vi "SeCrTs-DI Indexing.vi"(9 "data":T1={"AO config"=[], "AI config"=[], "DI config"=[], "DO config"=[], "TC config"=[], "ACC config"=[], "SG config"=[], "Strain Gauge Settings"={"poisson ratio"=0.3, "nominal gage resistance"=120.0, "gage factor"=2.08}, "Bridge Settings"={"voltage excitation value"=3.3, "voltage excitation source"=10200, "initial bridge voltage"=0.0, "lead wire resistance"=1.7, "strain configuration"=10271}, "Sample Rate"={"AI Sample Rate"=[], "AO Sample Rate"=[], "DI Sample Rate"=[], "TC Sample Rate"=[], "DO Sample Rate"=[], "SG Sample Rate"=[], "ACC Sample Rate"=[]}} {"Bridge Settings"."strain configuration" items=["Full Bridge I"=10183, "Full Bridge II"=10184, "Full Bridge III"=10185, "Half Bridge I"=10188, "Half Bridge II"=10189, "Quarter Bridge I"=10271, "Quarter Bridge II"=10272]; "Bridge Settings"."voltage excitation source" items=["Internal"=10200, "External"=10167, "None"=10230]; "ACC config"."Terminal configuration" items=["default"=-1, "RSE"=10083, "NRSE"=10078, "Differential"=10106, "Pseudodifferential"=12529]; "ACC config"."Sensitivity units" items=["mVolts/g"=12509, "Volts/g"=12510]; "TC config"."type" items=["J"=10072, "K"=10073, "N"=10077, "R"=10082, "S"=10085, "T"=10086, "B"=10047, "E"=10055]; "TC config"."units" items=["Deg C", "Deg F", "Kelvins", "Deg R", "From Custom Scale"]}) -> ()   [LabVIEW 2022 SP3]
uses:
  Controls/SeCrTs-Config.ctl
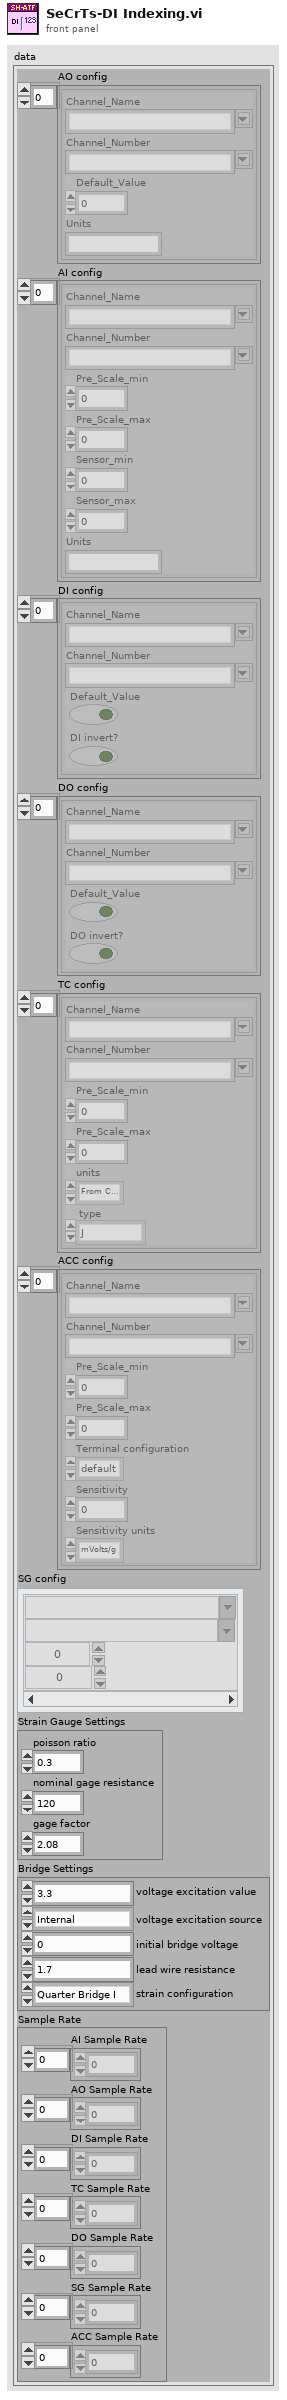
[diagram p1: front panel]
types:
  T1 = typedef "SeCrTs-Config.ctl" = cluster{"AO config":cluster{"Channel_Name":string, "Channel_Number":string, "Default_Value":dbl, "Units":string}[], "AI config":cluster{"Channel_Name":string, "Channel_Number":string, "Pre_Scale_min":dbl, "Pre_Scale_max":dbl, "Sensor_min":dbl, "Sensor_max":dbl, "Units":string}[], "DI config":cluster{"Channel_Name":string, "Channel_Number":string, "Default_Value":bool, "DI invert?":bool}[], "DO config":cluster{"Channel_Name":string, "Channel_Number":string, "Default_Value":bool, "DO invert?":bool}[], "TC config":cluster{"Channel_Name":string, "Channel_Number":string, "Pre_Scale_min":dbl, "Pre_Scale_max":dbl, "units":i32, " type":i32}[], "ACC config":cluster{"Channel_Name":string, "Channel_Number":string, "Pre_Scale_min":dbl, "Pre_Scale_max":dbl, "Terminal configuration":i32, "Sensitivity":dbl, "Sensitivity units":i32}[], "SG config":cluster{"Channel_Name":string, "Channel_Number":string, "Pre_Scale_min":dbl, "Pre_Scale_max":dbl}[], "Strain Gauge Settings":cluster{"poisson ratio":dbl, "nominal gage resistance":dbl, "gage factor":dbl}, "Bridge Settings":cluster{"voltage excitation value":dbl, "voltage excitation source":i32, "initial bridge voltage":dbl, "lead wire resistance":dbl, "strain configuration":i32}, "Sample Rate":cluster{"AI Sample Rate":dbl[], "AO Sample Rate":dbl[], "DI Sample Rate":dbl[], "TC Sample Rate":dbl[], "DO Sample Rate":dbl[], "SG Sample Rate":dbl[], "ACC Sample Rate":dbl[]}}
  T2 = cluster{"Channel_Name":string, "Channel_Number":string, "Default_Value":bool, "DI invert?":bool}[]
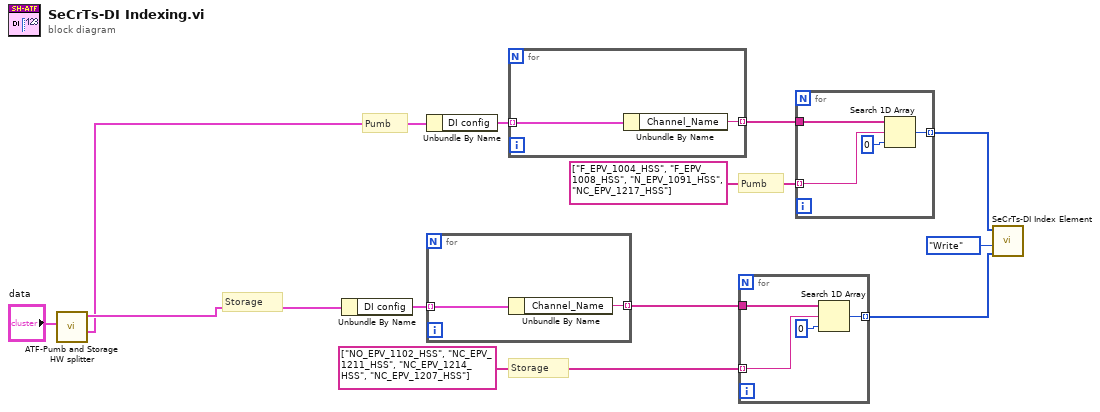
[diagram p0: block diagram]
diagram:
  # "Storage"
  # "Pumb"
  # "Pumb"
  # "Storage"
  n1 = call "ATF-Pumb and Storage HW splitter.vi"("data"="data") -> ("Pumb HW"=w3:T1, "Storage HW"=w4:T1)  [unwired: 9 in]
  n2 = Unbundle By Name(w4) -> ("DI config"=w1:T2)
  n3 = Unbundle By Name(w3) -> ("DI config"=w2:T2)
  n4 = for {
    tunnel: [w14] -> w12 mode=indexing
    tunnel: w1 -> [w13] mode=indexing
    n5 = Unbundle By Name(w13) -> ("Channel_Name"=w14:string)
  }
  n6 = for {
    tunnel: [w16] -> w8 mode=indexing
    tunnel: w2 -> [w15] mode=indexing
    n7 = Unbundle By Name(w15) -> ("Channel_Name"=w16:string)
  }
  n8 = for {
    tunnel: w12 -> [w20]
    tunnel: string[] ["NO_EPV_1102_HSS", "NC_EPV_1211_HSS", "NC_EPV_1214_HSS", "NC_EPV_1207_HSS"] -> [w19] mode=indexing
    tunnel: [w17] -> w9 mode=indexing
    n9 = Search 1D Array(1D array=w20, element=w19, start index (0)=0) -> (index of element=w17:i32)
  }
  n10 = for {
    tunnel: w8 -> [w24]
    tunnel: string[] ["F_EPV_1004_HSS", "F_EPV_1008_HSS", "N_EPV_1091_HSS", "NC_EPV_1217_HSS"] -> [w23] mode=indexing
    tunnel: [w21] -> w6 mode=indexing
    n11 = Search 1D Array(1D array=w24, element=w23, start index (0)=0) -> (index of element=w21:i32)
  }
  n12 = call "SeCrTs-DI Index Element.vi"("Storage Index"=w9, "Write/Read"=enum16{"Write", "Read"}."Write", "Pumb Index"=w6) -> ()  [unwired: 7 in, 2 out]
